vi "Trajectory Action to Robot Action.vi"(11 "Trajectory Action":T11) -> (3 "Robot Action":T1)   [LabVIEW 2019]
uses:
  Controls/Pivot Motor Commands.ctl
  Controls/Robot Drive Mode.ctl
  Controls/Robot Pivot Motion Commands.ctl
  Controls/Enable Actions.ctl
  Controls/Robot State.ctl
  Controls/Robot Actions.ctl
  Controls/Ball System Actions.ctl
  Controls/Spinner Actions.ctl
  Controls/Lift System Actions.ctl
  Controls/DriveJoystickData.ctl
  Controls/Trajectory Actions.ctl
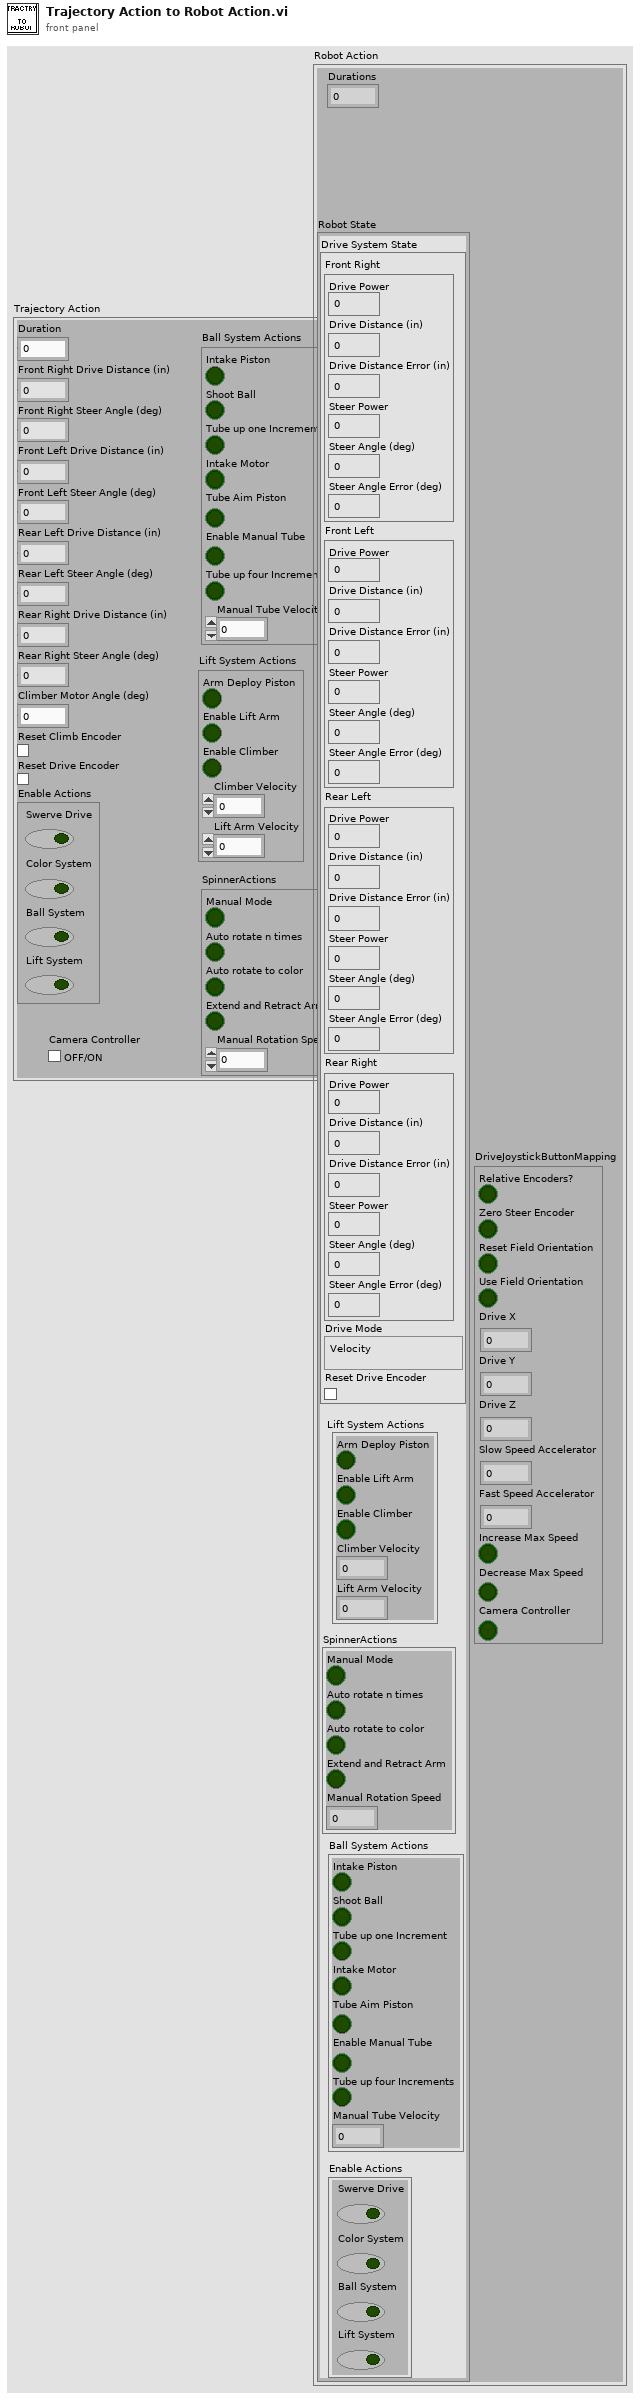
[diagram p1: front panel]
types:
  T1 = typedef "Robot Actions.ctl" = cluster{"Durations":dbl, "Robot State":T2, "DriveJoystickButtonMapping":T10}
  T2 = typedef "Robot State.ctl" = cluster{"Drive System State":T3, "Enable Actions":T6, "Lift System Actions":T7, "SpinnerActions":T8, "Ball System Actions":T9}
  T3 = typedef "Robot Pivot Motion Commands.ctl" = cluster{"Front Right":T4, "Front Left":T4, "Rear Left":T4, "Rear Right":T4, "Drive Mode":T5, "Reset Drive Encoder":bool}
  T4 = typedef "Pivot Motor Commands.ctl" = cluster{"Drive Power":dbl, "Drive Distance (in)":dbl, "Drive Distance Error (in)":dbl, "Steer Power":dbl, "Steer Angle (deg)":dbl, "Steer Angle Error (deg)":dbl}
  T5 = typedef "Robot Drive Mode.ctl" = enum16{"Velocity", "Distance"}
  T6 = typedef "Enable Actions.ctl" = cluster{"Swerve Drive":bool, "Color System":bool, "Ball System":bool, "Lift System":bool}
  T7 = typedef "Lift System Actions.ctl" = cluster{"Arm Deploy Piston":bool, "Enable Lift Arm":bool, "Enable Climber":bool, "Climber Velocity":dbl, "Lift Arm Velocity":dbl}
  T8 = typedef "Spinner Actions.ctl" = cluster{"Manual Mode ":bool, "Auto rotate n times":bool, "Auto rotate to color\t":bool, "Extend and Retract Arm\t":bool, "Manual Rotation Speed":dbl}
  T9 = typedef "Ball System Actions.ctl" = cluster{"Intake Piston ":bool, "Shoot Ball":bool, "Tube up one Increment\t":bool, "Intake Motor\t":bool, "Tube Aim Piston":bool, "Enable Manual Tube":bool, "Tube up four Increments":bool, "Manual Tube Velocity":dbl}
  T10 = typedef "DriveJoystickData.ctl" = cluster{"Relative Encoders?":bool, "Zero Steer Encoder":bool, "Reset Field Orientation":bool, "Use Field Orientation":bool, "Drive X":dbl, "Drive Y":dbl, "Drive Z":dbl, "Slow Speed Accelerator":dbl, "Fast Speed Accelerator":dbl, "Increase Max Speed":bool, "Decrease Max Speed":bool, "Camera Controller":bool}
  T11 = typedef "Trajectory Actions.ctl" = cluster{"Duration":dbl, "Front Right Drive Distance (in)":dbl, "Front Right Steer Angle (deg)":dbl, "Front Left Drive Distance (in)":dbl, "Front Left Steer Angle (deg)":dbl, "Rear Left Drive Distance (in)":dbl, "Rear Left Steer Angle (deg)":dbl, "Rear Right Drive Distance (in)":dbl, "Rear Right Steer Angle (deg)":dbl, "Climber Motor Angle (deg)":dbl, "Reset Climb Encoder":bool, "Reset Drive Encoder":bool, "Enable Actions":T6, "Lift System Actions":T7, "SpinnerActions":T8, "Ball System Actions":T9, "Camera Controller":bool}
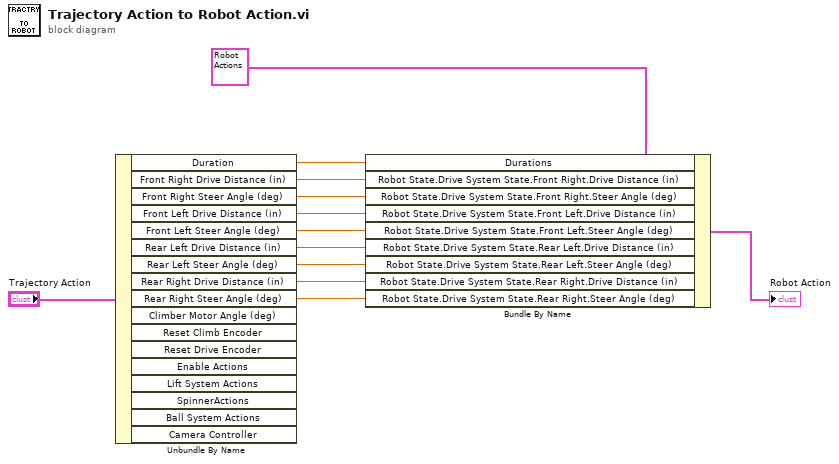
[diagram p0: block diagram]
diagram:
  n1 = Unbundle By Name("Trajectory Action") -> ("Duration"=w9:dbl, "Front Right Drive Distance (in)"=w8:dbl, "Front Right Steer Angle (deg)"=w7:dbl, "Front Left Drive Distance (in)"=w6:dbl, "Front Left Steer Angle (deg)"=w5:dbl, "Rear Left Drive Distance (in)"=w4:dbl, "Rear Left Steer Angle (deg)"=w3:dbl, "Rear Right Drive Distance (in)"=w2:dbl, "Rear Right Steer Angle (deg)"=w1:dbl)  [unwired: 8 out]
  n2 = Bundle By Name(cluster=T1 {"Durations"=0.0, "Robot State"={"Drive System State"={"Front Right"={"Drive Power"=0.0, "Drive Distance (in)"=0.0, "Drive Distance Error (in)"=0.0, "Steer Power"=0.0, "Steer Angle (deg)"=0.0, "Steer Angle Error (deg)"=0.0}, "Front Left"={"Drive Power"=0.0, "Drive Distance (in)"=0.0, "Drive Distance Error (in)"=0.0, "Steer Power"=0.0, "Steer Angle (deg)"=0.0, "Steer Angle Error (deg)"=0.0}, "Rear Left"={"Drive Power"=0.0, "Drive Distance (in)"=0.0, "Drive Distance Error (in)"=0.0, "Steer Power"=0.0, "Steer Angle (deg)"=0.0, "Steer Angle Error (deg)"=0.0}, "Rear Right"={"Drive Power"=0.0, "Drive Distance (in)"=0.0, "Drive Distance Error (in)"=0.0, "Steer Power"=0.0, "Steer Angle (deg)"=0.0, "Steer Angle Error (deg)"=0.0}, "Drive Mode"=enum."Velocity", "Reset Drive Encoder"=FALSE}, "Enable Actions"={"Swerve Drive"=FALSE, "Color System"=FALSE, "Ball System"=FALSE, "Lift System"=FALSE}, "Lift System Actions"={"Arm Deploy Piston"=FALSE, "Enable Lift Arm"=FALSE, "Enable Climber"=FALSE, "Climber Velocity"=0.0, "Lift Arm Velocity"=0.0}, "SpinnerActions"={"Manual Mode "=FALSE, "Auto rotate n times"=FALSE, "Auto rotate to color\t"=FALSE, "Extend and Retract Arm\t"=FALSE, "Manual Rotation Speed"=0.0}, "Ball System Actions"={"Intake Piston "=FALSE, "Shoot Ball"=FALSE, "Tube up one Increment\t"=FALSE, "Intake Motor\t"=FALSE, "Tube Aim Piston"=FALSE, "Enable Manual Tube"=FALSE, "Tube up four Increments"=FALSE, "Manual Tube Velocity"=0.0}}, "DriveJoystickButtonMapping"={"Relative Encoders?"=FALSE, "Zero Steer Encoder"=FALSE, "Reset Field Orientation"=FALSE, "Use Field Orientation"=FALSE, "Drive X"=0.0, "Drive Y"=0.0, "Drive Z"=0.0, "Slow Speed Accelerator"=0.0, "Fast Speed Accelerator"=0.0, "Increase Max Speed"=FALSE, "Decrease Max Speed"=FALSE, "Camera Controller"=FALSE}} ("Robot Action"), "Durations"=w9, "Robot State.Drive System State.Front Right.Drive Distance (in)"=w8, "Robot State.Drive System State.Front Right.Steer Angle (deg)"=w7, "Robot State.Drive System State.Front Left.Drive Distance (in)"=w6, "Robot State.Drive System State.Front Left.Steer Angle (deg)"=w5, "Robot State.Drive System State.Rear Left.Drive Distance (in)"=w4, "Robot State.Drive System State.Rear Left.Steer Angle (deg)"=w3, "Robot State.Drive System State.Rear Right.Drive Distance (in)"=w2, "Robot State.Drive System State.Rear Right.Steer Angle (deg)"=w1) -> (→"Robot Action":T1)
